vi "8-bit video export-setup format and update.vi"(11 "Array":T1[](array[typedef])) -> ()   [LabVIEW 2013]
uses:
  Typedefs/Image selector control.ctl
  Functional Imaging Viewer/Typedefs/Get-Set-Clear Control.ctl
  Cam video sync/Typedefs/Stitch layout spec cluster.ctl
  Typedefs/Image stitching positions.ctl
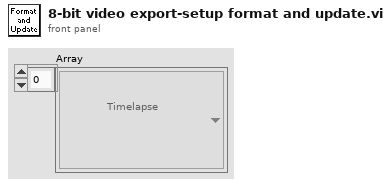
[diagram p1: front panel]
types:
  T1 = typedef "Image selector control.ctl" = enum16{"\n\nTimelapse", "\n\nVideo 1", "\n\nVideo 2", "\n\nVideo 3", "\n\nVideo 4", "\n\nNone"}
  T2 = typedef "Stitch layout spec cluster.ctl" = cluster{"Timelapse image":cluster{"Image position":T3}, "Cam 1":cluster{"Image position":T3}, "Cam 2":cluster{"Image position":T3}, "Cam 3":cluster{"Image position":T3}, "Cam 4":cluster{"Image position":T3}}
  T3 = typedef "Image stitching positions.ctl" = enum16{"Top left", "Top right", "Bottom left", "Bottom right", "Not used"}
  T4 = typedef "Get-Set-Clear Control.ctl" = enum16{"Get", "Set", "Clear"}
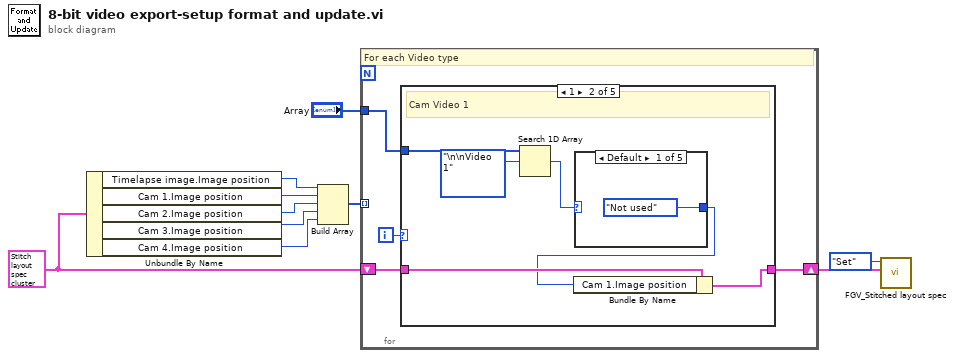
[diagram p0: block diagram]
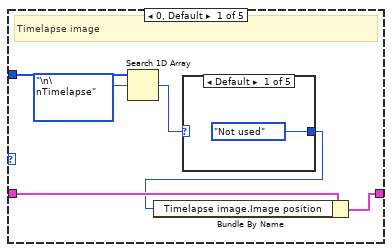
[diagram p2: hidden frame]
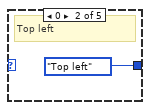
[diagram p3: hidden frame]
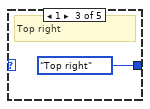
[diagram p4: hidden frame]
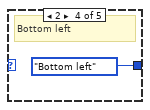
[diagram p5: hidden frame]
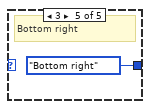
[diagram p6: hidden frame]
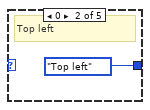
[diagram p7: hidden frame]
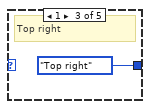
[diagram p8: hidden frame]
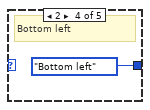
[diagram p9: hidden frame]
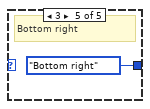
[diagram p10: hidden frame]
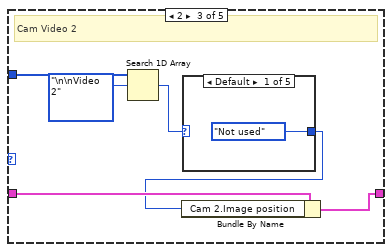
[diagram p11: hidden frame]
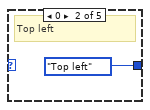
[diagram p12: hidden frame]
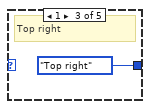
[diagram p13: hidden frame]
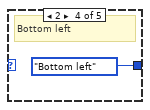
[diagram p14: hidden frame]
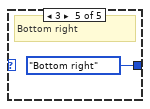
[diagram p15: hidden frame]
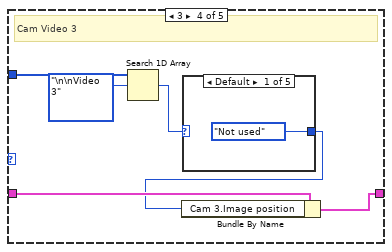
[diagram p16: hidden frame]
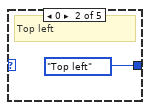
[diagram p17: hidden frame]
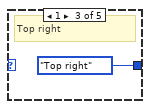
[diagram p18: hidden frame]
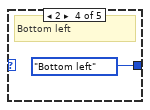
[diagram p19: hidden frame]
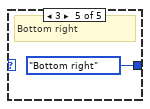
[diagram p20: hidden frame]
diagram:
  w10 = T2 {"Timelapse image"={"Image position"=enum."Not used"}, "Cam 1"={"Image position"=enum."Not used"}, "Cam 2"={"Image position"=enum."Not used"}, "Cam 3"={"Image position"=enum."Not used"}, "Cam 4"={"Image position"=enum."Not used"}} ("Stitch layout spec")
  n1 = Unbundle By Name(w10) -> ("Timelapse image.Image position"=w3:T3, "Cam 1.Image position"=w4:T3, "Cam 2.Image position"=w5:T3, "Cam 3.Image position"=w6:T3, "Cam 4.Image position"=w7:T3)
  n2 = Build Array(w3, w4, w5, w6, w7) -> (w8:T3[])
  n3 = for {
    shift-right: [w12] -> w2
    shift-left: w10 -> [w13]
    tunnel: w8 -> [_] mode=indexing
    tunnel: "Array" -> [w11]
    i -> [w14]
    # "For each Video type"
    n4 = case shown="1" w14 {
      tunnel: w13 -> [w20 w31 w42 w53 w64]
      tunnel: [w19 w30 w41 w52 w63] -> w12
      tunnel: w11 -> [w18 w29 w40 w51 w62]
      frame 0, Default {
        # "Timelapse image"
        n5 = Search 1D Array(1D array=w18, element=Image_selector_control."\n\nTimelapse" ("Top left")) -> (index of element=w16:i32)  [unwired: 1 in]
        n6 = case shown="Default" w16 {
          tunnel: [Image_stitching_positions."Not used" ("Timelapse image.Image position") Image_stitching_positions."Top left" ("Timelapse image.Image position") Image_stitching_positions."Top right" ("Timelapse image.Image position") Image_stitching_positions."Bottom left" ("Timelapse image.Image position") Image_stitching_positions."Bottom right" ("Timelapse image.Image position")] -> w15
          frame Default {
          }
          frame 0 {
            # "Top left"
          }
          frame 1 {
            # "Top right"
          }
          frame 2 {
            # "Bottom left"
          }
          frame 3 {
            # "Bottom right"
          }
        }
        n7 = Bundle By Name(cluster=w20, "Timelapse image.Image position"=w15) -> (w19:T2)
      }
      frame 1 {
        # "Cam Video 1"
        n8 = Search 1D Array(1D array=w29, element=Image_selector_control."\n\nVideo 1" ("Top left")) -> (index of element=w27:i32)  [unwired: 1 in]
        n9 = case shown="Default" w27 {
          tunnel: [Image_stitching_positions."Not used" ("Timelapse image.Image position") Image_stitching_positions."Top left" ("Timelapse image.Image position") Image_stitching_positions."Top right" ("Timelapse image.Image position") Image_stitching_positions."Bottom left" ("Timelapse image.Image position") Image_stitching_positions."Bottom right" ("Timelapse image.Image position")] -> w26
          frame Default {
          }
          frame 0 {
            # "Top left"
          }
          frame 1 {
            # "Top right"
          }
          frame 2 {
            # "Bottom left"
          }
          frame 3 {
            # "Bottom right"
          }
        }
        n10 = Bundle By Name(cluster=w31, "Cam 1.Image position"=w26) -> (w30:T2)
      }
      frame 2 {
        # "Cam Video 2"
        n11 = Search 1D Array(1D array=w40, element=Image_selector_control."\n\nVideo 2" ("Top left")) -> (index of element=w38:i32)  [unwired: 1 in]
        n12 = case shown="Default" w38 {
          tunnel: [Image_stitching_positions."Not used" ("Timelapse image.Image position") Image_stitching_positions."Top left" ("Timelapse image.Image position") Image_stitching_positions."Top right" ("Timelapse image.Image position") Image_stitching_positions."Bottom left" ("Timelapse image.Image position") Image_stitching_positions."Bottom right" ("Timelapse image.Image position")] -> w37
          frame Default {
          }
          frame 0 {
            # "Top left"
          }
          frame 1 {
            # "Top right"
          }
          frame 2 {
            # "Bottom left"
          }
          frame 3 {
            # "Bottom right"
          }
        }
        n13 = Bundle By Name(cluster=w42, "Cam 2.Image position"=w37) -> (w41:T2)
      }
      frame 3 {
        # "Cam Video 3"
        n14 = Search 1D Array(1D array=w51, element=Image_selector_control."\n\nVideo 3" ("Top left")) -> (index of element=w49:i32)  [unwired: 1 in]
        n15 = case shown="Default" w49 {
          tunnel: [Image_stitching_positions."Not used" ("Timelapse image.Image position") Image_stitching_positions."Top left" ("Timelapse image.Image position") Image_stitching_positions."Top right" ("Timelapse image.Image position") Image_stitching_positions."Bottom left" ("Timelapse image.Image position") Image_stitching_positions."Bottom right" ("Timelapse image.Image position")] -> w48
          frame Default {
          }
          frame 0 {
            # "Top left"
          }
          frame 1 {
            # "Top right"
          }
          frame 2 {
            # "Bottom left"
          }
          frame 3 {
            # "Bottom right"
          }
        }
        n16 = Bundle By Name(cluster=w53, "Cam 3.Image position"=w48) -> (w52:T2)
      }
      frame 4 {
        # "Cam Video 4"
        n17 = Search 1D Array(1D array=w62, element=Image_selector_control."\n\nVideo 4" ("Top left")) -> (index of element=w60:i32)  [unwired: 1 in]
        n18 = case shown="Default" w60 {
          tunnel: [Image_stitching_positions."Not used" ("Timelapse image.Image position") Image_stitching_positions."Top left" ("Timelapse image.Image position") Image_stitching_positions."Top right" ("Timelapse image.Image position") Image_stitching_positions."Bottom left" ("Timelapse image.Image position") Image_stitching_positions."Bottom right" ("Timelapse image.Image position")] -> w59
          frame Default {
          }
          frame 0 {
            # "Top left"
          }
          frame 1 {
            # "Top right"
          }
          frame 2 {
            # "Bottom left"
          }
          frame 3 {
            # "Bottom right"
          }
        }
        n19 = Bundle By Name(cluster=w64, "Cam 4.Image position"=w59) -> (w63:T2)
      }
    }
  }
  n20 = call "FGV_Stitched layout spec.vi"("Stitch layout spec"=w2, "Function"=Get-Set-Clear_Control."Set") -> ()  [unwired: 8 in, 2 out]
